vi "Internal Message Queue - Close.vi"(8 "error in (no error)":errorcluster, 11 "Plugin in":refnum<class "Generic Plugin.lvclass">) -> (0 "error out":errorcluster, 3 "Plugin out":refnum<class "Generic Plugin.lvclass">)   [LabVIEW 2020, in "RxnRover.lvlib" / "Generic Plugin.lvclass"]
doc: "Close the internal message queue of the plugin server."
uses:
  Generic Plugin.lvclass
  Generic Plugin.lvclass/Generic Plugin.ctl
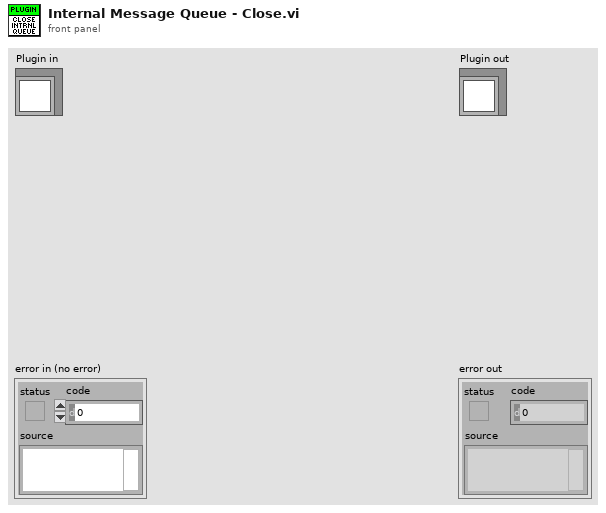
[diagram p1: front panel]
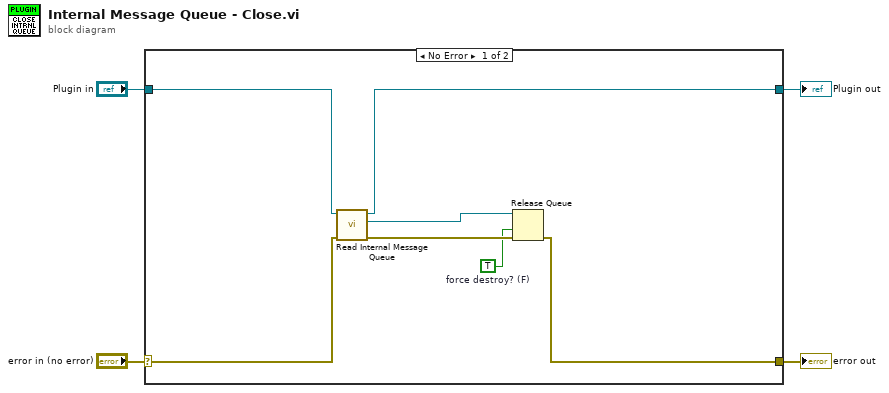
[diagram p0: block diagram]
diagram:
  n1 = case shown="No Error" "error in (no error)" {
    selector: "error in (no error)" -> [w11 w13]
    tunnel: [w6 w13] -> w3
    tunnel: [w7 w12] -> w1
    tunnel: "Plugin in" -> [w10 w12]
    frame No Error {
      w5 = TRUE  # force destroy? (F)
      n2 = call "Read Internal Message Queue.vi"("error in (no error)"=w11, "Generic Controller in"=w10) -> ("error out"=w8:errorcluster, "Internal Message Queue"=w9:refnum<queue>, "Generic Controller out"=w7:refnum<class "Generic Plugin.lvclass">)  [unwired: 7 in]
      n3 = Release Queue(queue=w9, force destroy? (F)=w5, error in (no error)=w8) -> (error out=w6:errorcluster)  [unwired: 2 out]
    }
    frame Error {
    }
  }
  "error out" <- w3
  "Plugin out" <- w1
